vi "Barcodeprint.vi"() -> ()   [LabVIEW 2020]
uses:
  System.Drawing
  BarcodeLib.dll
  Sources/Global_Variable/Global.vi
panel:
  out "error out":errorcluster
  in  "错误输入（无错误）":errorcluster
  in  "保存位置":string="D:\\"
  in  "二维码颜色":u32(colorbox)
  in  "背景颜色":u32(colorbox)=16777215
  in  "单选按钮":enum32{"保存", "打印"}(radio)=enum."打印"
  in  "包含条形码标签":bool
  out "二维码图片":picture
  in  "高度":i32=200
  in  "宽度":i32=700
  in  "保存类型":i32(ring)=2 items=["JPG", "BMP", "PNG", "GIF", "TIFF", "UNSPECIFIED"]
  in  "编码类型":i32(ring)=27 items=["UNSPECIFIED", "UPCA", "UPCE", "UPC_SUPPLEMENTAL_2DIGIT", "UPC_SUPPLEMENTAL_5DIGIT", "EAN13", "EAN8", "Interleaved2of5", "Standard2of5", "Industrial2of5", "CODE39", "CODE39Extended", "Codabar", "PostNet", "BOOKLAND", "ISBN", "JAN13", "MSI_Mod10", "MSI_2Mod10", "MSI_Mod11", "MSI_Mod11_Mod10", "Modified_Plessey", "CODE11", "USD8", "UCC12", "UCC13", "LOGMARS", "CODE128", "CODE128A", "CODE128B", "CODE128C", "ITF14", "CODE93", "TELEPEN", "FIM"]
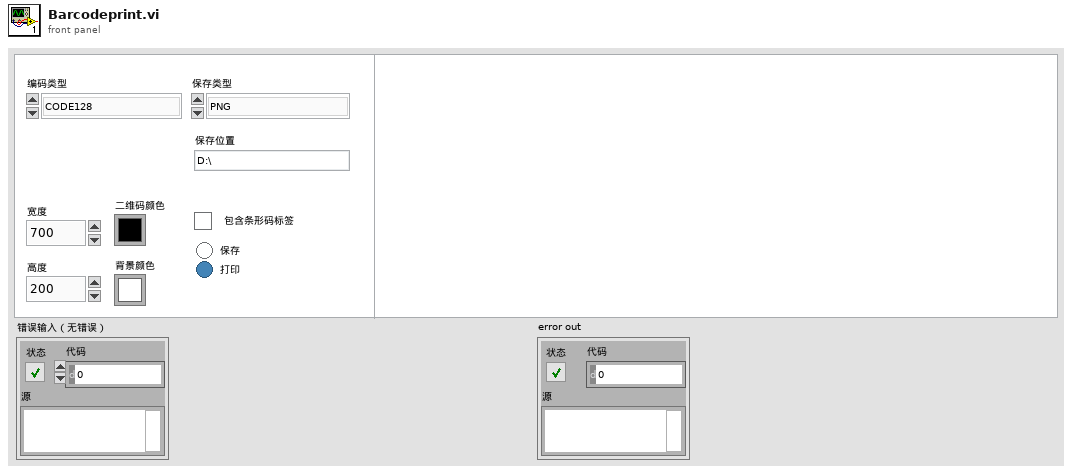
[diagram p1: front panel]
types:
  T1 = typedef "imagedata.ctl" = cluster{"image type":i32, "image depth":i32, "image":u8[], "mask":u8[], "colors":u32[], "Rectangle":cluster{"left":i16, "top":i16, "right":i16, "bottom":i16}}
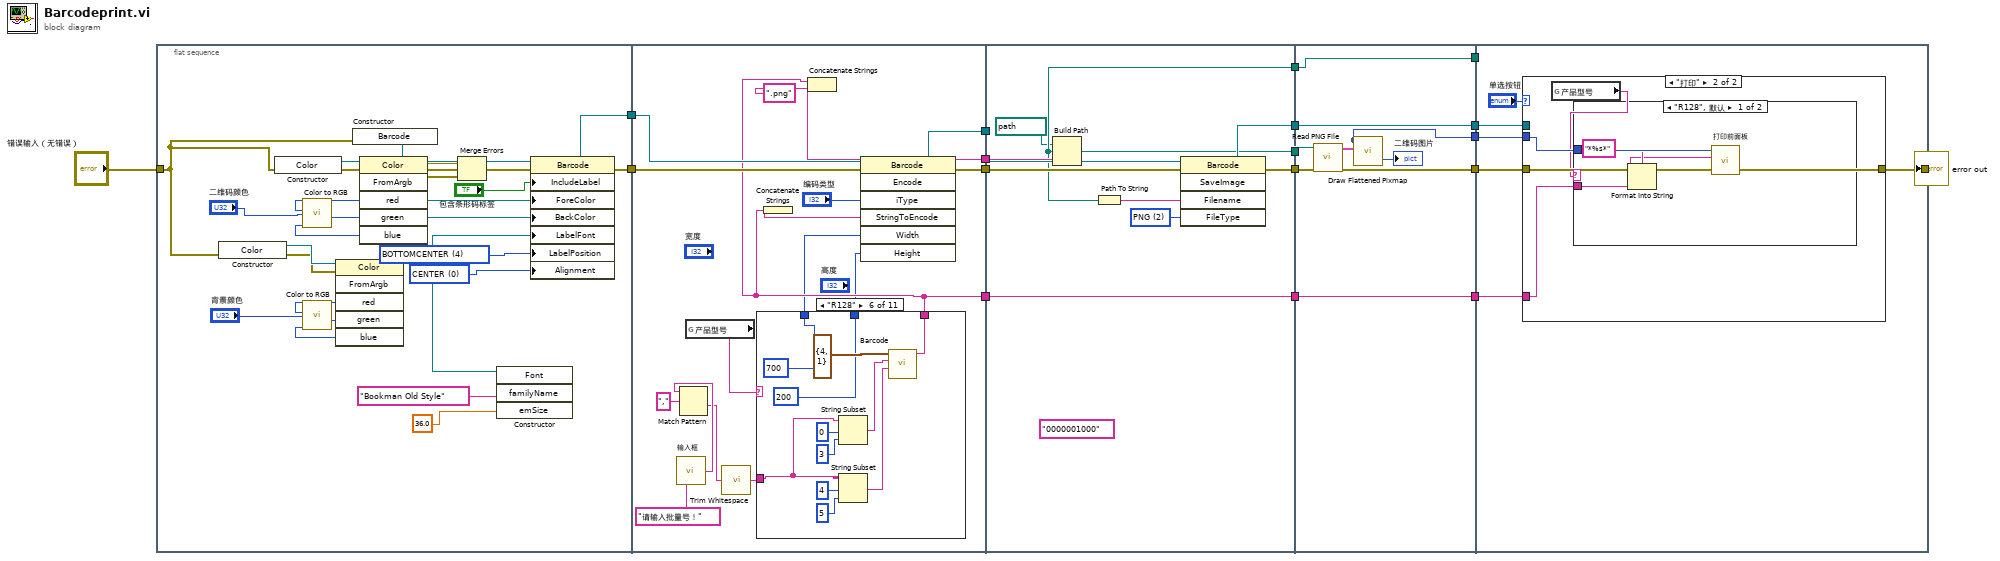
[diagram p0: block diagram]
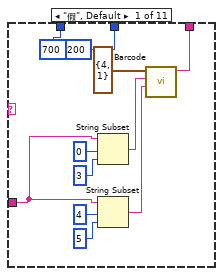
[diagram p2: hidden frame]
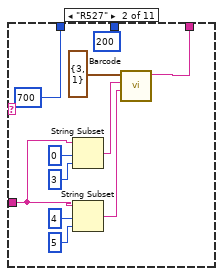
[diagram p3: hidden frame]
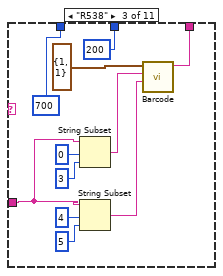
[diagram p4: hidden frame]
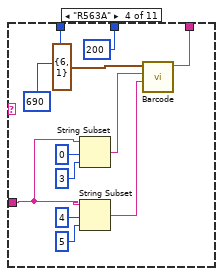
[diagram p5: hidden frame]
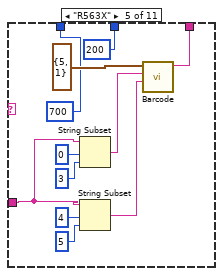
[diagram p6: hidden frame]
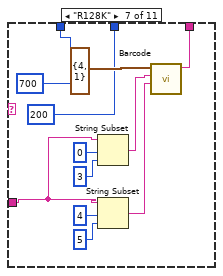
[diagram p7: hidden frame]
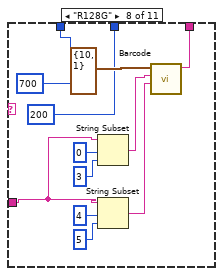
[diagram p8: hidden frame]
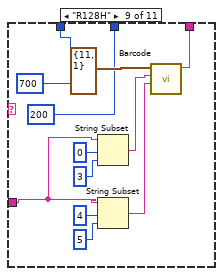
[diagram p9: hidden frame]
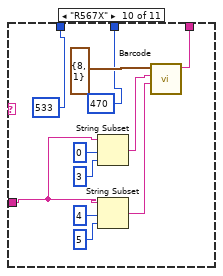
[diagram p10: hidden frame]
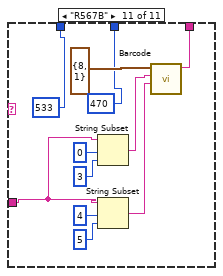
[diagram p11: hidden frame]
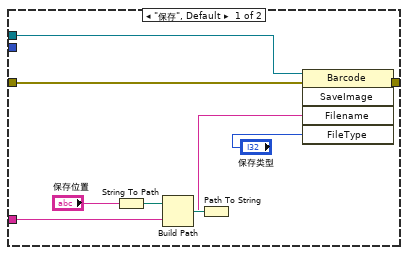
[diagram p12: hidden frame]
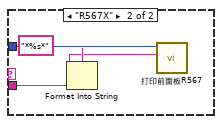
[diagram p13: hidden frame]
diagram:
  n1 = flat-sequence {
    tunnel: [w45] -> w18
    tunnel: [w44] -> w17
    tunnel: "错误输入（无错误）" -> [w24]
    tunnel: w18 -> [w62]
    tunnel: w17 -> [w61]
    tunnel: [w60] -> w16
    tunnel: [w59] -> w15
    tunnel: [w57] -> w14
    tunnel: [w55] -> w1
    tunnel: w16 -> [w194]
    tunnel: w15 -> [w193]
    tunnel: w14 -> [w189]
    tunnel: [w191] -> w13
    tunnel: [w190] -> w12
    tunnel: [w187] -> w11
    tunnel: [w185] -> w7
    tunnel: [w187] -> w5
    tunnel: w1 -> [w185]
    tunnel: w13 -> [w202]
    tunnel: w12 -> [w197]
    tunnel: w11 -> [w200]
    tunnel: [w202] -> w10
    tunnel: [w196] -> w9
    tunnel: [w199] -> w8
    tunnel: w7 -> [w199]
    tunnel: [w198] -> w6
    tunnel: w5 -> [w198]
    tunnel: [w195] -> w2
    tunnel: w10 -> [w207]
    tunnel: w9 -> [w206]
    tunnel: w8 -> [w205]
    tunnel: w6 -> [_]
    tunnel: [w204] -> w3
    tunnel: w2 -> [w203]
    frame #0 {
      w19 = 0 items=["CENTER", "LEFT", "RIGHT"] ("Alignment")
      w20 = 4 items=["TOPLEFT", "TOPCENTER", "TOPRIGHT", "BOTTOMLEFT", "BOTTOMCENTER", "BOTTOMRIGHT"] ("LabelPosition")
      n2 = constructor class="Color"(error in=w24) -> (reference out=w36:refnum<k24>, error out=w29:errorcluster)  [unwired: 2 in, 1 out]
      n3 = constructor class="Color"(error in=w24) -> (reference out=w38:refnum<k24>, error out=w30:errorcluster)  [unwired: 2 in, 1 out]
      n4 = call <vilib>:"Color to RGB.vi"("Color"="二维码颜色") -> ("R"=w41:u8, "G"=w40:u8, "B"=w39:u8)  [unwired: 1 out]
      n5 = call <vilib>:"Color to RGB.vi"("Color"="背景颜色") -> ("R"=w33:u8, "G"=w34:u8, "B"=w35:u8)  [unwired: 1 out]
      n6 = invoke class="Color" method="FromArgb"(reference=w36, error in=w29, "red"=w33, "green"=w34, "blue"=w35) -> (error out=w26:errorcluster, "FromArgb"=w32:refnum<k24>)  [unwired: 1 in, 4 out]
      n7 = constructor class="Barcode"(error in=w24) -> (reference out=w46:refnum<k24>, error out=w27:errorcluster)  [unwired: 2 in, 1 out]
      n8 = invoke class="Color" method="FromArgb"(reference=w38, error in=w30, "red"=w41, "green"=w40, "blue"=w39) -> (error out=w28:errorcluster, "FromArgb"=w37:refnum<k24>)  [unwired: 1 in, 4 out]
      n9 = Merge Errors(w27, w28, w26) -> (w25:errorcluster)
      n10 = constructor class="Font"("familyName"="Bookman Old Style", "emSize"=sgl 36.0) -> (reference out=w21:refnum<k24>)  [unwired: 3 in, 4 out]
      n11 = property on="属性节点" class="Barcode"(reference=w46, error in=w25, "IncludeLabel"="包含条形码标签", "ForeColor"=w37, "BackColor"=w32, "LabelFont"=w21, "LabelPosition"=w20, "Alignment"=w19) -> (reference out=w45:refnum<k24>, error out=w44:errorcluster)
    }
    frame #1 {
      n12 = call "输入框.vi"("提示信息"="请输入批量号！") -> ("条形码输出"=w50:string)
      n13 = Match Pattern(string=w50, regular expression="," ("正则表达式")) -> (after substring=w49:string)  [unwired: 1 in, 3 out]
      n14 = global read "Global.vi" "产品型号"() -> (w54:string)
      n15 = call <vilib>:"Trim Whitespace.vi"("string"=w49) -> ("trimmed string"=w52:string)  [unwired: 1 in]
      n16 = case shown="\"R128\"" w54 {
        tunnel: [w68 w85 w95 w106 w117 w128 w139 w150 w161 w172 w183] -> w55
        tunnel: w52 -> [w66 w79 w90 w101 w112 w123 w134 w145 w156 w167 w178]
        tunnel: [700 ("start row") 700 ("start row") 700 ("start row") 690 ("start column") 700 ("start row") 700 ("start row") 700 ("start row") 700 ("start row") 700 ("start row") 533 ("start row") 533 ("start row")] -> w48
        tunnel: [200 ("start row") 200 ("start row") 200 ("start row") 200 ("start row") 200 ("start row") 200 ("start row") 200 ("start row") 200 ("start row") 200 ("start row") 470 ("start row") 470 ("start row")] -> w47
        frame "假", Default {
          n17 = String Subset(string=w66, offset (0)=0 ("偏移量(0)"), length (rest)=3 ("长度（剩余）")) -> (substring=w74:string)
          n18 = String Subset(string=w66, offset (0)=4 ("偏移量(0)"), length (rest)=5 ("长度（剩余）")) -> (substring=w73:string)
          n19 = call "Barcode.vi"("流水号"=w73, "年月日"=w74, "start (0, 0)"=cluster{"start row":i32, "start column":i32} {"start row"=4, "start column"=1}) -> ("条形码"=w68:string)  [unwired: 8 in]
        }
        frame "R527" {
          n20 = String Subset(string=w79, offset (0)=0 ("偏移量(0)"), length (rest)=3 ("长度（剩余）")) -> (substring=w78:string)
          n21 = String Subset(string=w79, offset (0)=4 ("偏移量(0)"), length (rest)=5 ("长度（剩余）")) -> (substring=w77:string)
          n22 = call "Barcode.vi"("流水号"=w77, "年月日"=w78, "start (0, 0)"=cluster{"start row":i32, "start column":i32} {"start row"=3, "start column"=1}) -> ("条形码"=w85:string)  [unwired: 8 in]
        }
        frame "R538" {
          n23 = String Subset(string=w90, offset (0)=0 ("偏移量(0)"), length (rest)=3 ("长度（剩余）")) -> (substring=w89:string)
          n24 = String Subset(string=w90, offset (0)=4 ("偏移量(0)"), length (rest)=5 ("长度（剩余）")) -> (substring=w88:string)
          n25 = call "Barcode.vi"("流水号"=w88, "年月日"=w89, "start (0, 0)"=cluster{"start row":i32, "start column":i32} {"start row"=1, "start column"=1}) -> ("条形码"=w95:string)  [unwired: 8 in]
        }
        frame "R563A" {
          n26 = String Subset(string=w101, offset (0)=0 ("偏移量(0)"), length (rest)=3 ("长度（剩余）")) -> (substring=w100:string)
          n27 = String Subset(string=w101, offset (0)=4 ("偏移量(0)"), length (rest)=5 ("长度（剩余）")) -> (substring=w99:string)
          n28 = call "Barcode.vi"("流水号"=w99, "年月日"=w100, "start (0, 0)"=cluster{"start row":i32, "start column":i32} {"start row"=6, "start column"=1}) -> ("条形码"=w106:string)  [unwired: 8 in]
        }
        frame "R563X" {
          n29 = String Subset(string=w112, offset (0)=0 ("偏移量(0)"), length (rest)=3 ("长度（剩余）")) -> (substring=w111:string)
          n30 = String Subset(string=w112, offset (0)=4 ("偏移量(0)"), length (rest)=5 ("长度（剩余）")) -> (substring=w110:string)
          n31 = call "Barcode.vi"("流水号"=w110, "年月日"=w111, "start (0, 0)"=cluster{"start row":i32, "start column":i32} {"start row"=5, "start column"=1}) -> ("条形码"=w117:string)  [unwired: 8 in]
        }
        frame "R128" {
          n32 = String Subset(string=w123, offset (0)=0 ("偏移量(0)"), length (rest)=3 ("长度（剩余）")) -> (substring=w122:string)
          n33 = String Subset(string=w123, offset (0)=4 ("偏移量(0)"), length (rest)=5 ("长度（剩余）")) -> (substring=w121:string)
          n34 = call "Barcode.vi"("流水号"=w121, "年月日"=w122, "start (0, 0)"=cluster{"start row":i32, "start column":i32} {"start row"=4, "start column"=1}) -> ("条形码"=w128:string)  [unwired: 8 in]
        }
        frame "R128K" {
          n35 = String Subset(string=w134, offset (0)=0 ("偏移量(0)"), length (rest)=3 ("长度（剩余）")) -> (substring=w133:string)
          n36 = String Subset(string=w134, offset (0)=4 ("偏移量(0)"), length (rest)=5 ("长度（剩余）")) -> (substring=w132:string)
          n37 = call "Barcode.vi"("流水号"=w132, "年月日"=w133, "start (0, 0)"=cluster{"start row":i32, "start column":i32} {"start row"=4, "start column"=1}) -> ("条形码"=w139:string)  [unwired: 8 in]
        }
        frame "R128G" {
          n38 = String Subset(string=w145, offset (0)=0 ("偏移量(0)"), length (rest)=3 ("长度（剩余）")) -> (substring=w144:string)
          n39 = String Subset(string=w145, offset (0)=4 ("偏移量(0)"), length (rest)=5 ("长度（剩余）")) -> (substring=w143:string)
          n40 = call "Barcode.vi"("流水号"=w143, "年月日"=w144, "start (0, 0)"=cluster{"start row":i32, "start column":i32} {"start row"=10, "start column"=1}) -> ("条形码"=w150:string)  [unwired: 8 in]
        }
        frame "R128H" {
          n41 = String Subset(string=w156, offset (0)=0 ("偏移量(0)"), length (rest)=3 ("长度（剩余）")) -> (substring=w155:string)
          n42 = String Subset(string=w156, offset (0)=4 ("偏移量(0)"), length (rest)=5 ("长度（剩余）")) -> (substring=w154:string)
          n43 = call "Barcode.vi"("流水号"=w154, "年月日"=w155, "start (0, 0)"=cluster{"start row":i32, "start column":i32} {"start row"=11, "start column"=1}) -> ("条形码"=w161:string)  [unwired: 8 in]
        }
        frame "R567X" {
          n44 = String Subset(string=w167, offset (0)=0 ("偏移量(0)"), length (rest)=3 ("长度（剩余）")) -> (substring=w166:string)
          n45 = String Subset(string=w167, offset (0)=4 ("偏移量(0)"), length (rest)=5 ("长度（剩余）")) -> (substring=w165:string)
          n46 = call "Barcode.vi"("流水号"=w165, "年月日"=w166, "start (0, 0)"=cluster{"start row":i32, "start column":i32} {"start row"=8, "start column"=1}) -> ("条形码"=w172:string)  [unwired: 8 in]
        }
        frame "R567B" {
          n47 = String Subset(string=w178, offset (0)=0 ("偏移量(0)"), length (rest)=3 ("长度（剩余）")) -> (substring=w177:string)
          n48 = String Subset(string=w178, offset (0)=4 ("偏移量(0)"), length (rest)=5 ("长度（剩余）")) -> (substring=w176:string)
          n49 = call "Barcode.vi"("流水号"=w176, "年月日"=w177, "start (0, 0)"=cluster{"start row":i32, "start column":i32} {"start row"=8, "start column"=1}) -> ("条形码"=w183:string)  [unwired: 8 in]
        }
      }
      n50 = Concatenate Strings(w55) -> (w56:string)
      n51 = Concatenate Strings(w55, ".png" ("字符串")) -> (w57:string)
      n52 = invoke class="Barcode" method="Encode"(reference=w62, error in=w61, "iType"="编码类型", "StringToEncode"=w56, "Width"=w48, "Height"=w47) -> (reference out=w60:refnum<k24>, error out=w59:errorcluster)  [unwired: 1 in, 5 out]
    }
    frame #2 {
      (unwired) "0000001000" ("条形码")
      w192 = 2 items=["JPG", "BMP", "PNG", "GIF", "TIFF", "UNSPECIFIED"] ("FileType")
      n53 = Build Path(base path=path "D:/条码" ("基路径"), name or relative path=w189) -> (appended path=w187:path)
      n54 = Path To String(path=w187) -> (string=w188:string)
      n55 = invoke class="Barcode" method="SaveImage"(reference=w194, error in=w193, "Filename"=w188, "FileType"=w192) -> (reference out=w191:refnum<k24>, error out=w190:errorcluster)  [unwired: 1 in, 3 out]
    }
    frame #3 {
      n56 = call <vilib>:"Read PNG File.vi"("error in (no error)"=w197, "path to PNG file"=w200) -> ("error out"=w196:errorcluster, "image data"=w201:T1)  [unwired: 7 in, 1 out]
      n57 = call <vilib>:"Draw Flattened Pixmap.vi"("image data"=w201) -> ("new picture"=w195:picture)  [unwired: 8 in]
      "二维码图片" <- w195
    }
    frame #4 {
      n58 = case shown="\"打印\"" "单选按钮" {
        tunnel: w207 -> [w217 _]
        tunnel: w206 -> [w216 w220]
        tunnel: w205 -> [w210 w219]
        tunnel: [w209 w220] -> w204
        tunnel: w203 -> [_ w221]
        frame "保存", Default {
          n59 = String To Path(string="保存位置") -> (path=w214:path)
          n60 = Build Path(base path=w214, name or relative path=w210) -> (appended path=w215:path)
          n61 = Path To String(path=w215) -> (string=w212:string)
          n62 = invoke class="Barcode" method="SaveImage"(reference=w217, error in=w216, "Filename"=w212, "FileType"="保存类型") -> (error out=w209:errorcluster)  [unwired: 1 in, 4 out]
        }
        frame "打印" {
          n63 = global read "Global.vi" "产品型号"() -> (w218:string)
          n64 = case shown="\"R128\", 默认" w218 {
            tunnel: w221 -> [w225 w229]
            tunnel: w219 -> [w223 w227]
            frame "R128", Default {
              n65 = Format Into String(format string="*%s*" ("格式字符串"), w223) -> (resulting string=w222:string)  [unwired: 2 in, 1 out]
              n66 = call "打印前面板.vi"("字符串"=w222, "二维码图片"=w225) -> ()  [unwired: 10 in]
            }
            frame "R567X" {
              n67 = Format Into String(format string="*%s*" ("格式字符串"), w227) -> (resulting string=w226:string)  [unwired: 2 in, 1 out]
              n68 = call "打印前面板R567.vi"("字符串"=w226, "二维码图片"=w229) -> ()  [unwired: 10 in]
            }
          }
        }
      }
    }
  }
  "error out" <- w3
